vi "Get Sample Style Atributes.vi"(2 "StyleNumRef":refnum<vi>) -> (0 "SampleSpecs":T1)   [LabVIEW 2015]
panel:
  out "error OUT":errorcluster
  in  "error IN":errorcluster
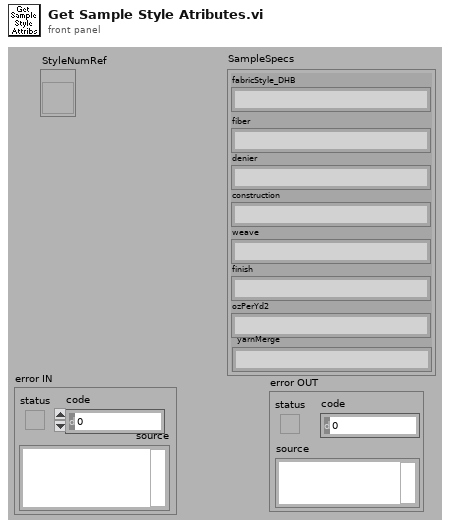
[diagram p1: front panel]
types:
  T1 = cluster{"fiber":string, "denier":string, "construction":string, "weave":string, "finish":string, "ozPerYd2":string, "fabricStyle_DHB":string, "yarnMerge":string}
  T2 = cluster{"recordset data[0]":string, "recordset data[1]":string, "recordset data[2]":string, "recordset data[3]":string, "recordset data[4]":string, "recordset data[5]":string, "recordset data[6]":string, "recordset data[7]":string}
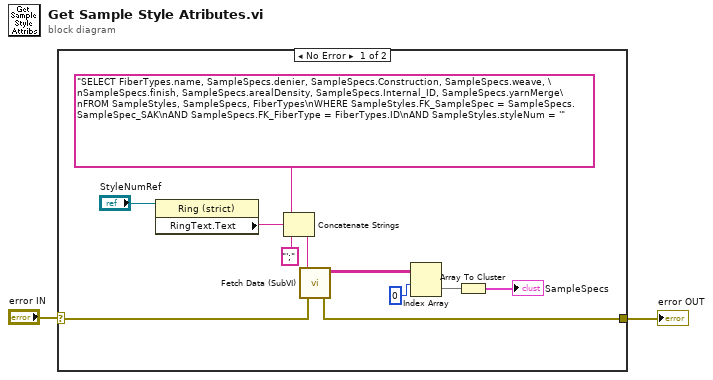
[diagram p0: block diagram]
diagram:
  n1 = case shown="No Error" "error IN" {
    selector: "error IN" -> [w4 w14]
    tunnel: [w3 w14] -> w1
    frame No Error {
      n2 = property on="Property Node" class="Ring (strict)"(reference="StyleNumRef") -> ("RingText.Text"=w6:string)  [unwired: 1 in, 2 out]
      n3 = Concatenate Strings("SELECT FiberTypes.name, SampleSpecs.denier, SampleSpecs.Construction, SampleSpecs.weave, \nSampleSpecs.finish, SampleSpecs.arealDensity, SampleSpecs.Internal_ID, SampleSpecs.yarnMerge\nFROM SampleStyles, SampleSpecs, FiberTypes\nWHERE SampleStyles.FK_SampleSpec = SampleSpecs.SampleSpec_SAK\nAND SampleSpecs.FK_FiberType = FiberTypes.ID\nAND SampleStyles.styleNum = '", w6, "';" ("string")) -> (w8:string)
      n4 = call "Fetch Data (SubVI).vi"("error IN"=w4, "query string"=w8) -> ("error OUT"=w3:errorcluster, "recordset data"=w13:string[][])  [unwired: 4 out]
      n5 = Index Array(array=w13, index (row)=0 ("disabled index (col)")) -> (element=w5:string[])  [unwired: 1 in]
      n6 = Array To Cluster(array=w5) -> (cluster=→"SampleSpecs":T2)
    }
    frame Error {
    }
  }
  "error OUT" <- w1
